vi "TCP Write com tamanho.vi"(0 "connection ID":refnum<k5>, 2 "data in":string, 5 "error in (no error)":errorcluster) -> (14 "connection out":refnum<k5>, 19 "error out":errorcluster)   [LabVIEW 2012]
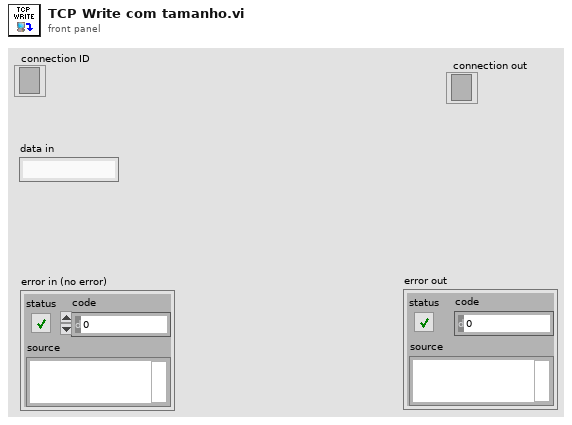
[diagram p1: front panel]
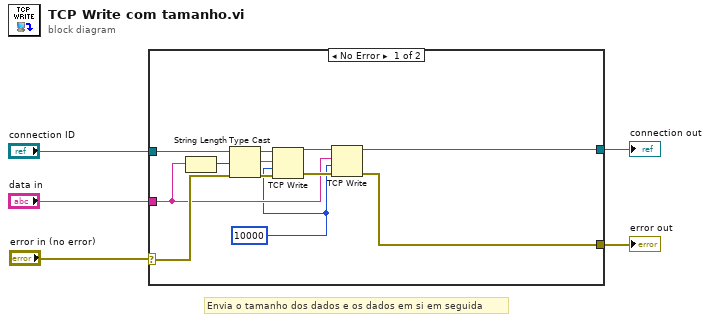
[diagram p0: block diagram]
diagram:
  # "Envia o tamanho dos dados e os dados em si em seguida"
  n1 = case shown="No Error" "error in (no error)" {
    selector: "error in (no error)" -> [w14 w16]
    tunnel: "connection ID" -> [w15 w17]
    tunnel: [w11 w16] -> w3
    tunnel: [w10 w17] -> w2
    tunnel: "data in" -> [w7 _]
    frame No Error {
      w6 = 10000 ("timeout ms (25000)")
      n2 = String Length(string=w7) -> (length=w9:i32)
      n3 = Type Cast(x=w9) -> (*(type *) &x=w8:string)  [unwired: 1 in]
      n4 = TCP Write(connection ID=w15, data in=w8, error in (no error)=w14, 9:w6) -> (connection ID out=w13:refnum<k5>, error out=w12:errorcluster)  [unwired: 1 out]
      n5 = TCP Write(connection ID=w13, data in=w7, error in (no error)=w12, 9:w6) -> (connection ID out=w10:refnum<k5>, error out=w11:errorcluster)  [unwired: 1 out]
    }
    frame Error {
    }
  }
  "error out" <- w3
  "connection out" <- w2
